vi "RT Driver VI.vi"(7 "Operation":T1, 11 "Device Reference in":T2 format="%.0x") -> (0 "Error Code":i32)   [LabVIEW 2023, in "Vires VTD Engine.lvlib"]
uses:
  Vires VTD Engine.lvlib
  <vilib>/NI VeriStand/Custom Device API/Custom Device Item Ref.ctl
  <vilib>/NI VeriStand/Custom Device API/Hardware Interface Driver VI Operation.ctl
  Shared/Compiled.Settings.ctl
  System Explorer/RDB Data.ctl
  RDB/RDB Object.ctl
  RDB/RDB Player Object.ctl
  Shared/Network Settings.ctl
  Shared/Protocol.ctl
  Shared/SensorInfos.ctl
  Shared/SensorInfo.ctl
  Shared/Sensor Name.ctl
  MM/MM Data.ctl
  MM/MM Objects.ctl
  MM/MM Object.ctl
  Shared/Timedloop Settings.ctl
  Type/RTStateVariables.ctl
  <vilib>/NI/NIVS Inline Async API/_VS Inline Async API/VS Inline Async API/VS Inline Async API.lvclass
  <vilib>/NI/NIVS Inline Async API/_VS Inline Async API/VS Inline Async API/VS Inline Async API.lvclass/VS Inline Async API.ctl
  <vilib>/NI/NIVS Inline Async API/_Data Access Engine/Data Access Engine/Data Access Engine.lvclass/Data Access Engine.ctl
  <vilib>/NI/NIVS Inline Async API/_Data Access Engine/Access Type Classes/Write/Write.lvclass/Write.ctl
  <vilib>/NI/NIVS Inline Async API/_Data Access Engine/Access Type Classes/ReadWrite/ReadWrite.lvclass/ReadWrite.ctl
  <vilib>/NI/NIVS Inline Async API/_Data Access Engine/Access Type Classes/Read/Read.lvclass/Read.ctl
  <vilib>/NI/NIVS Inline Async API/_Data Access Engine/Data Access Engine/Methods/Data.Engine.Read Data from HW.vi
  <vilib>/NI/NIVS Inline Async API/_VS Inline Async API/Error Handling Process/SubVIs/Error.GetError.vi
  <vilib>/NI/NIVS Inline Async API/_Data Access Engine/Data Access Engine/Methods/Data.Engine.Write Data to HW.vi
  <vilib>/NI/NIVS Inline Async API/_Data Access Engine/Access Type Classes/ReadWrite/ReadWrite.EngineData.vi
  <vilib>/NI/NIVS Inline Async API/_Data Access Engine/Access Type Classes/Write/Write.EngineData.vi
  <vilib>/NI/NIVS Inline Async API/_Data Access Engine/Access Type Classes/Read/Read.EngineData.vi
  <vilib>/NI VeriStand/Custom Device API/NI VeriStand - Get Channel Value by Data Reference.vi
  <vilib>/NI VeriStand/Custom Device API/NI VeriStand - Set Channel Value by Data Reference.vi
  <vilib>/NI VeriStand/Custom Device API/NI VeriStand - Get Channel Values by Block Data Reference.vi
  ModuleManager.vi
  <vilib>/NI VeriStand/Custom Device API/Get Item Property (Variant).vi
  <vilib>/NI VeriStand/Custom Device API/Global Data Refs.vi
  <vilib>/NI VeriStand/Custom Device API/Custom Device API.lvlib
  <vilib>/NI VeriStand/Custom Device Tools/Custom Device Utility Library/Custom Device Utility Library.lvlib
  Shared/Vires VTD Shared.lvlib
  RDB/RDB.lvlib
  MM/MM.lvlib
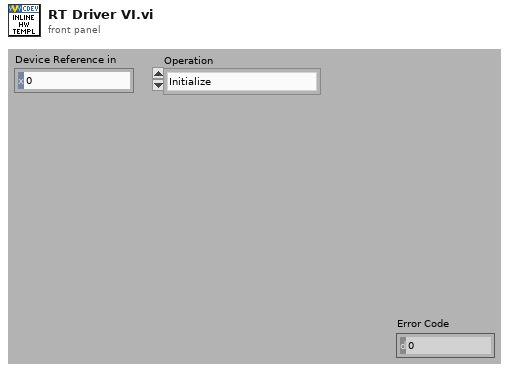
[diagram p1: front panel]
types:
  T1 = typedef "Custom Device API.lvlib/Hardware Interface Driver VI Operation.ctl" = enum16{"Initialize", "Start", "Read Data from HW", "Write Data to HW", "Close"}
  T2 = typedef "Custom Device API.lvlib/Custom Device Item Ref.ctl" = u64
  T3 = typedef "Vires VTD Engine.lvlib/RTStateVariables.ctl" = cluster{"Async":refnum<class "VS Inline Async API.lvclass">, "Settings":T4}
  T4 = typedef "Vires VTD Shared.lvlib/Compiled.Settings.ctl" = cluster{"Name":string, "RDB Data Receive ":T5, "RDB Data Sent":T5, "vclient":path, "Network Settings":T8, "SensorInfos":T10, "mmanager":path, "Scenario Paths":string[], "Custom SCP Commands":string[], "Timed Loop Settings for TaskControl":T16, "Timed Loop Settings for ModuleManager":T16}
  T5 = typedef "Vires VTD Shared.lvlib/RDB Data.ctl" = T6[]
  T6 = typedef "RDB.lvlib/RDB Object.ctl" = cluster{"pkID":i32, "RDB Player Objects":T7[]}
  T7 = typedef "RDB.lvlib/RDB Player Object.ctl" = cluster{"PlayerID":i32, "Signals":string[], "adv para":i32}
  T8 = typedef "Vires VTD Shared.lvlib/Network Settings.ctl" = cluster{"IP adress":string, "RDB":cluster{"Protocol":T9, "Tx Port":u16, "Rx Port":u16, "Buffer Size":i32, "Timeout":u16}, "SCP":cluster{"Protocol":T9, "Tx Port":u16, "Rx Port":u16, "Buffer Size":i32, "Timeout":u16}}
  T9 = typedef "Vires VTD Shared.lvlib/Protocol.ctl" = enum16{"UDP", "TCP"}
  T10 = typedef "Vires VTD Shared.lvlib/SensorInfos.ctl" = T11[]
  T11 = typedef "Vires VTD Shared.lvlib/SensorInfo.ctl" = cluster{"Sensor Name":T12, "Protocol":T9, "Network port":i32, "# Culled Objects":i32, "PlayerID":u8, "MM Data":T13}
  T12 = typedef "Vires VTD Shared.lvlib/Sensor Name.ctl" = string
  T13 = typedef "Vires VTD Shared.lvlib/MM Data.ctl" = T14[]
  T14 = typedef "MM.lvlib/MM Objects.ctl" = cluster{"pkID":i32, "MM Objects":T15[]}
  T15 = typedef "MM.lvlib/MM Object.ctl" = cluster{"Object":i32, "Signals":string[]}
  T16 = typedef "Vires VTD Shared.lvlib/Timedloop Settings.ctl" = cluster{"Period(ms)":i64, "Priority":i32, "Processor":i32}
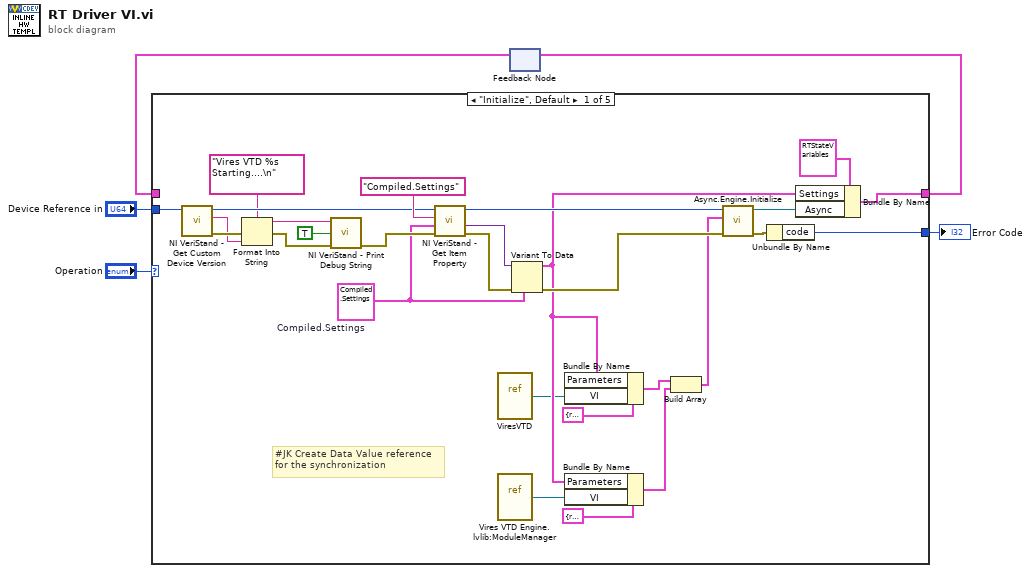
[diagram p0: block diagram]
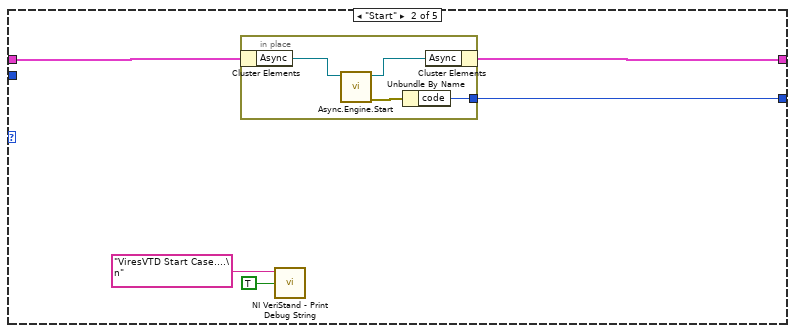
[diagram p2: hidden frame]
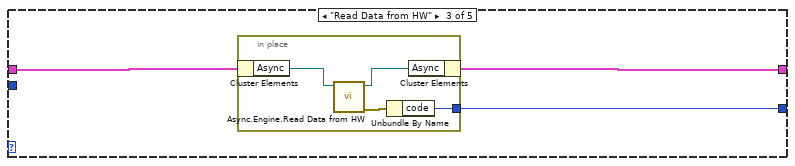
[diagram p3: hidden frame]
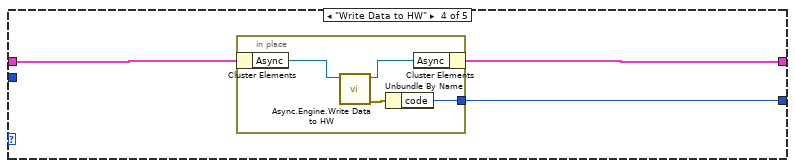
[diagram p4: hidden frame]
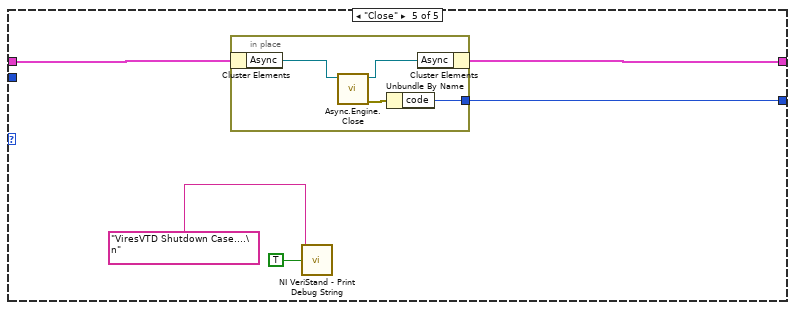
[diagram p5: hidden frame]
diagram:
  n1 = feedback #1() -> (w3:T3)  [unwired: 1 out]
  n2 = case shown="\"Initialize\", Default" "Operation" {
    tunnel: [w32 w37 w43 w50 w60] -> w4
    tunnel: w3 -> [_ w38 w45 w51 w61]
    tunnel: "Device Reference in" -> [w18 _ _ _ _]
    tunnel: [w33 w36 w44 w52 w59] -> w1
    frame "Initialize", Default {
      w27 = T4 {"Name"="", "RDB Data Receive "=[], "RDB Data Sent"=[], "vclient"=path "", "Network Settings"={"IP adress"="127.0.0.1", "RDB"={"Protocol"=enum."UDP", "Tx Port"=10, "Rx Port"=10, "Buffer Size"=204800, "Timeout"=10}, "SCP"={"Protocol"=enum."TCP", "Tx Port"=48191, "Rx Port"=48191, "Buffer Size"=204800, "Timeout"=10}}, "SensorInfos"=[], "mmanager"=path "", "Scenario Paths"=[], "Custom SCP Commands"=[], "Timed Loop Settings for TaskControl"={"Period(ms)"=2, "Priority"=100, "Processor"=-2}, "Timed Loop Settings for ModuleManager"={"Period(ms)"=2, "Priority"=100, "Processor"=-2}}  # Compiled.Settings
      # "#JK Create Data Value reference\nfor the synchronization"
      n3 = call <vilib>:"NI VeriStand - Get Custom Device Version.vi"("Device Ref in"=w18) -> ("error out"=w16:errorcluster, "Value"=w15:string, "Device Ref out"=w17:T2)  [unwired: 8 in]
      n4 = Format Into String(format string="Vires VTD %s Starting....\n" ("Message"), error in=w16, w15) -> (resulting string=w13:string, error out=w14:errorcluster)  [unwired: 1 in]
      n5 = call <vilib>:"NI VeriStand - Print Debug String.vi"("error in (no error)"=w14, "Add to log file? (F)"=TRUE ("Add to log file? (T)"), "Message"=w13) -> ("error out"=w28:errorcluster)  [unwired: 8 in]
      n6 = call-poly <vilib>:"NI VeriStand - Get Item Property.vi"("error in (no error)"=w28, "Default Value"=w27, "Property Name"="Compiled.Settings", "Item Ref in"=w17) -> ("error out"=w31:errorcluster, "Value"=w30:variant, "Item Ref out"=w23:T2)  [unwired: 4 in, 1 out]
      n7 = vi-ref "ViresVTD.vi"() -> (w7:refnum<vi>)
      n8 = vi-ref "Vires VTD Engine.lvlib:ModuleManager.vi"() -> (w10:refnum<vi>)
      n9 = Variant To Data(error in=w31, type=w27, Variant=w30) -> (data=w20:T4, error out=w25:errorcluster)
      n10 = Bundle By Name(cluster=cluster{"VI":refnum<vi>, "Parameters":variant} {"VI"=refnum, "Parameters"=variant} ("Process"), "Parameters"=w20, "VI"=w7) -> (w6:cluster{"VI":refnum<vi>, "Parameters":variant})
      n11 = Bundle By Name(cluster=cluster{"VI":refnum<vi>, "Parameters":variant} {"VI"=refnum, "Parameters"=variant} ("Process"), "Parameters"=w20, "VI"=w10) -> (w9:cluster{"VI":refnum<vi>, "Parameters":variant})
      n12 = Build Array(w6, w9) -> (w24:cluster{"VI":refnum<vi>, "Parameters":variant}[])
      n13 = call <vilib>:"Async.Engine.Initialize.vi"("error in (no error)"=w25, "Processes"=w24, "Custom Device Ref"=w23) -> ("error out"=w21:errorcluster, "Async"=w22:refnum<class "VS Inline Async API.lvclass">)  [unwired: 7 in]
      n14 = Unbundle By Name(w21) -> ("code"=w33:i32)
      n15 = Bundle By Name(cluster=T3 {"Async"=refnum, "Settings"={"Name"="", "RDB Data Receive "=[], "RDB Data Sent"=[], "vclient"=path "", "Network Settings"={"IP adress"="127.0.0.1", "RDB"={"Protocol"=enum."UDP", "Tx Port"=10, "Rx Port"=10, "Buffer Size"=204800, "Timeout"=10}, "SCP"={"Protocol"=enum."TCP", "Tx Port"=48191, "Rx Port"=48191, "Buffer Size"=204800, "Timeout"=10}}, "SensorInfos"=[], "mmanager"=path "", "Scenario Paths"=[], "Custom SCP Commands"=[], "Timed Loop Settings for TaskControl"={"Period(ms)"=2, "Priority"=100, "Processor"=-2}, "Timed Loop Settings for ModuleManager"={"Period(ms)"=2, "Priority"=100, "Processor"=-2}}} ("RT State Variables"), "Settings"=w20, "Async"=w22) -> (w32:T3)
    }
    frame "Start" {
      n16 = in-place {
        in-place-border: [w39] -> w36
        n17 = in-place-cluster #2(w38) -> ("Async"=w42:refnum<class "VS Inline Async API.lvclass">)
        n18 = call <vilib>:"Async.Engine.Start.vi"("VS Inline Async API in"=w42) -> ("error out"=w40:errorcluster, "VS Inline Async API out"=w41:refnum<class "VS Inline Async API.lvclass">)  [unwired: 9 in]
        n19 = Unbundle By Name(w40) -> ("code"=w39:i32)
        n20 = in-place-cluster #2("Async"=w41) -> (w37:T3)
      }
      n21 = call <vilib>:"NI VeriStand - Print Debug String.vi"("Add to log file? (F)"=TRUE ("Add to log file? (T)"), "Message"="ViresVTD Start Case....\n") -> ()  [unwired: 9 in, 1 out]
    }
    frame "Read Data from HW" {
      n22 = in-place {
        in-place-border: [w47] -> w44
        n23 = in-place-cluster #3(w45) -> ("Async"=w49:refnum<class "VS Inline Async API.lvclass">)
        n24 = call <vilib>:"Async.Engine.Read Data from HW.vi"("Async in"=w49) -> ("error out"=w46:errorcluster, "Async out"=w48:refnum<class "VS Inline Async API.lvclass">)  [unwired: 9 in]
        n25 = Unbundle By Name(w46) -> ("code"=w47:i32)
        n26 = in-place-cluster #3("Async"=w48) -> (w43:T3)
      }
    }
    frame "Write Data to HW" {
      n27 = in-place {
        in-place-border: [w56] -> w52
        n28 = in-place-cluster #4(w51) -> ("Async"=w54:refnum<class "VS Inline Async API.lvclass">)
        n29 = call <vilib>:"Async.Engine.Write Data to HW.vi"("VS Inline Async API in"=w54) -> ("error out"=w55:errorcluster, "VS Inline Async API out"=w53:refnum<class "VS Inline Async API.lvclass">)  [unwired: 9 in]
        n30 = Unbundle By Name(w55) -> ("code"=w56:i32)
        n31 = in-place-cluster #4("Async"=w53) -> (w50:T3)
      }
    }
    frame "Close" {
      n32 = in-place {
        in-place-border: [w63] -> w59
        n33 = in-place-cluster #5(w61) -> ("Async"=w65:refnum<class "VS Inline Async API.lvclass">)
        n34 = call <vilib>:"Async.Engine.Close.vi"("Async in"=w65) -> ("error out"=w62:errorcluster, "Async out"=w64:refnum<class "VS Inline Async API.lvclass">)  [unwired: 9 in]
        n35 = Unbundle By Name(w62) -> ("code"=w63:i32)
        n36 = in-place-cluster #5("Async"=w64) -> (w60:T3)
      }
      n37 = call <vilib>:"NI VeriStand - Print Debug String.vi"("Add to log file? (F)"=TRUE ("Add to log file? (T)"), "Message"="ViresVTD Shutdown Case....\n") -> ()  [unwired: 9 in, 1 out]
    }
  }
  "Error Code" <- w1
  n38 = feedback-in #1(w4) -> ()
